vi "Line Circle Intersection.vi"(8 "error in (no error)":errorcluster, 9 "Circle Center":cluster{"x":dbl, "y":dbl}={"x"=2.0, "y"=0.0}, 10 "Line's Angle (rads)":dbl, 11 "Circle Radius":dbl=1.0) -> (0 "error out":errorcluster, 2 "Intersection?":bool, 3 "Points of Intersection":cluster{dbl, dbl}[](array[cluster]))   [LabVIEW 2011]
uses:
  <vilib>/Analysis/polynomials.llb/Polynomial Roots (DBL).vi
  <vilib>/Analysis/NI_AALPro.lvlib
panel:
  out "Y Values":dbl[](array[numeric])
  out "Coefficients for P(x)":dbl[](array[numeric])
  out "slope (m)":dbl
  out "X values of intersection":cdb[](array[numeric])
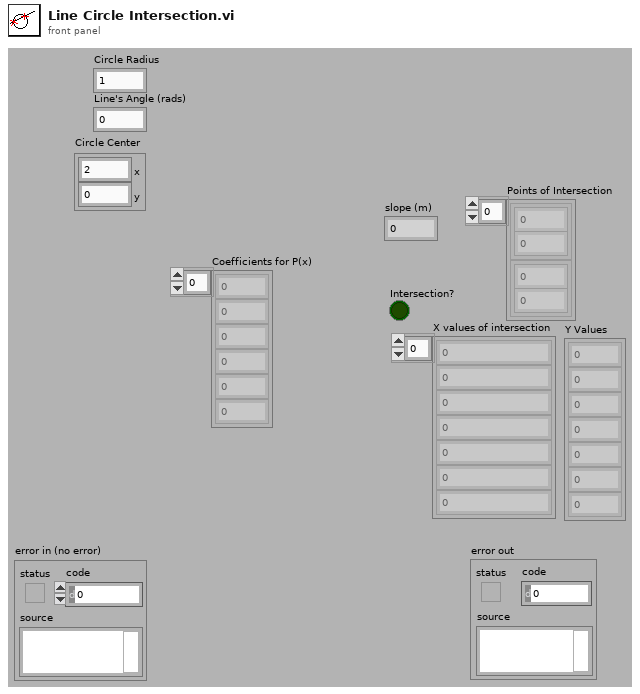
[diagram p1: front panel]
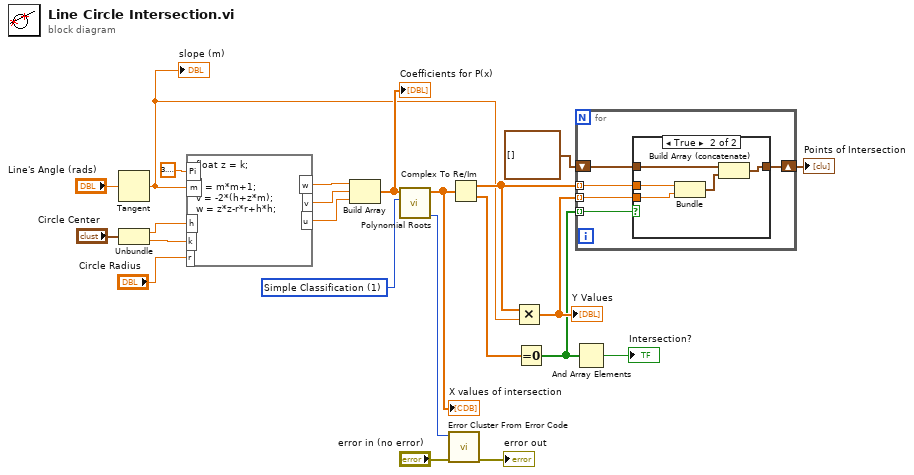
[diagram p0: block diagram]
diagram:
  w19 = u16 1 items=["General", "Simple Classification", "Refinement", "Advanced Refinement"] ("option")
  n1 = Tangent(1:"Line's Angle (rads)") -> (0:w2:dbl)
  "slope (m)" <- w2
  n2 = Unbundle("Circle Center") -> ("x"=w16:dbl, "y"=w15:dbl)
  n3 = formula code="float z = k;\n\nu = m*m+1;\nv = -2*(h+z*m);\nw = z*z-r*r+h*h;"("m"=w2, "h"=w16, "r"="Circle Radius", "k"=w15, "Pi"=3.141592653589793) -> ("u"=w23:dbl, "v"=w22:dbl, "w"=w21:dbl)
  n4 = Build Array(w21, w22, w23) -> (w20:dbl[])
  "Coefficients for P(x)" <- w20
  n5 = call-poly <vilib>:"Polynomial Roots.vi"("option"=w19, "P(x)"=w20) -> ("error"=w6:i32, "Roots"=w13:cdb[])  [unwired: 8 out]
  "X values of intersection" <- w13
  n6 = call <vilib>:"Error Cluster From Error Code.vi"("error in (no error)"="error in (no error)", "error code (0)"=w6) -> ("error out"=→"error out":errorcluster)  [unwired: 7 in]
  n7 = Complex To Re/Im(x + iy=w13) -> (x=w7:dbl[], y=w12:dbl[])
  n8 = Multiply(x=w7, y=w2) -> (x*y=w14:dbl[])
  "Y Values" <- w14
  n9 = Equal To 0?(x=w12) -> (x = 0?=w10:bool[])
  n10 = for {
    tunnel: w14 -> [w27] mode=indexing
    tunnel: w7 -> [w28] mode=indexing
    tunnel: w10 -> [w26] mode=indexing
    shift-right: [w24] -> w11
    shift-left: cluster{dbl, dbl}[] [] ("initialized array") -> [w25]
    n11 = case shown="True" w26 {
      tunnel: w28 -> [_ w34]
      tunnel: w27 -> [_ w33]
      tunnel: w25 -> [w29 w31]
      tunnel: [w29 w32] -> w24
      frame False {
      }
      frame True {
        n12 = Bundle(w34, w33) -> (w30:cluster{dbl, dbl})  [unwired: 1 out]
        n13 = Build Array (concatenate)(w31, w30) -> (w32:cluster{dbl, dbl}[])
      }
    }
  }
  "Points of Intersection" <- w11
  n14 = And Array Elements(Boolean array=w10) -> (logical AND=→"Intersection?":bool)
